vi "Host.vi"() -> ()   [LabVIEW 2025]
uses:
  <vilib>/FPGAPlugInAG/cRIO-9033/niLvFpga_Open_cRIO-9033.vi
  <vilib>/rvi/interface/common/dynamic/niFpgaDynamicAddResources.vi
  <vilib>/FPGAPlugInAG/Dynamic/niLvFpga_Reset_Dynamic.vi
  <vilib>/Utility/error.llb/Error Cluster From Error Code.vi
  <vilib>/rvi/errors/niLvFpgaAdjustHostInterfaceError.vi
  <vilib>/FPGAPlugInAG/Dynamic/niLvFpga_Run_Dynamic.vi
  <vilib>/FPGAPlugInAG/Dynamic/niLvFpga_Close_Dynamic.vi
  <vilib>/rvi/interface/nirviOpenFPGA/nirviOpenFPGA.xnode
  FPGA Bitfiles/parallelhmmlponf_FPGATarget_Target4_-PQN8YsI7Fc.lvbitx
  Target4.vi
  <vilib>/rvi/interface/nirviMethod/nirviMethod.xnode
  <vilib>/rvi/interface/nirviCloseFPGA/nirviCloseFPGA.xnode
  <vilib>/rvi/errors/niLvFpgaMergeErrorWithErrorCode.vi
  <vilib>/FPGAPlugInAG/Dynamic/niLvFpga_ReadFifo_Dynamic.vi
  <vilib>/FPGAPlugInAG/Dynamic/niLvFpga_WriteFifo_Dynamic.vi
panel:
  out "Window(s)":dbl[][](array[numeric])
  out "input":dbl[][](array[numeric])
  out "Healthy%":sgl[](array[numeric])
  out "Unhealthy%":sgl[](array[numeric])
  out "Timing":u32[](array[numeric])
  out "size(s)":i32[](array[numeric])
  out "Uncontrolled Acceleration":dynamicdata(graph)
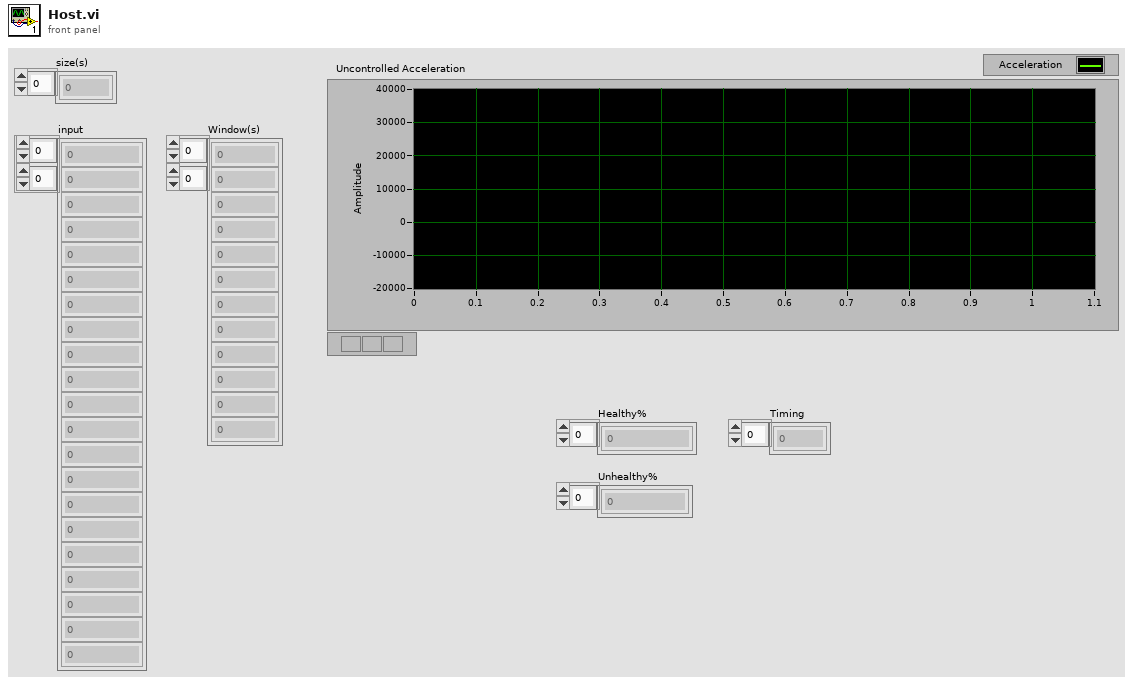
[diagram p1: front panel]
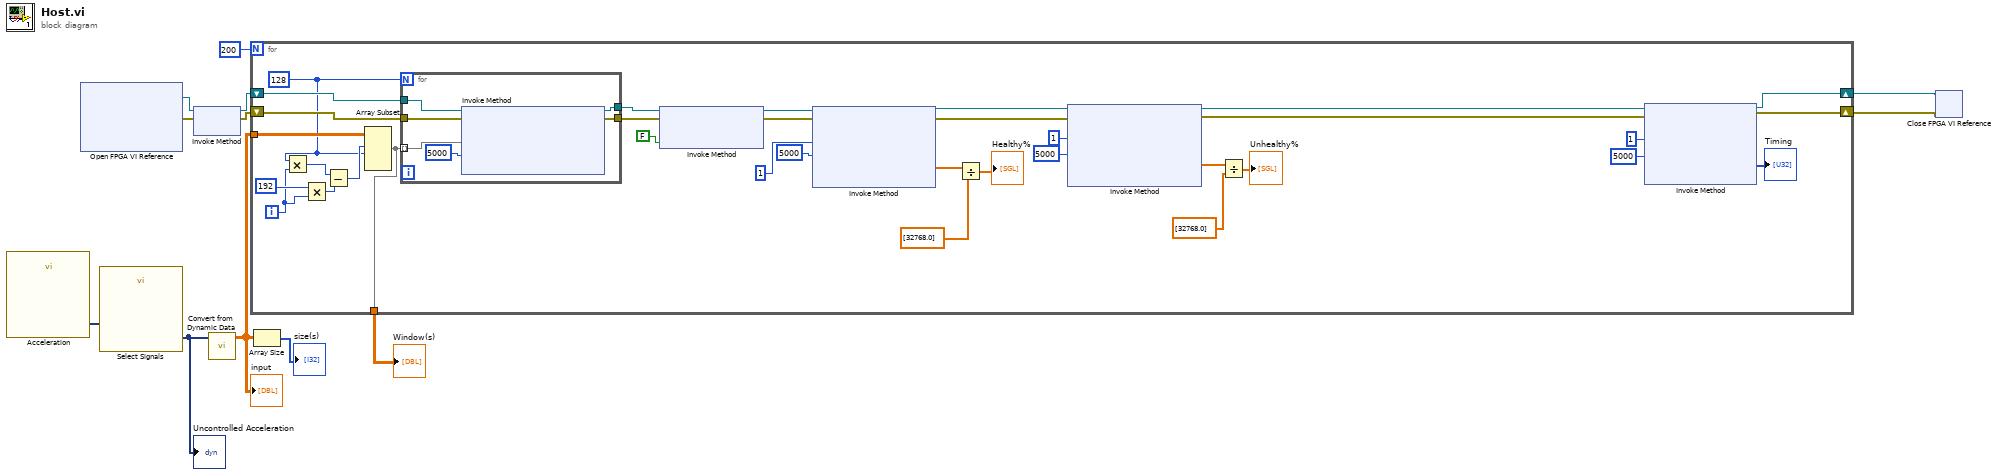
[diagram p0: block diagram]
diagram:
  n1 = call "Acceleration"() -> ("Signals"=w12:dynamicdata)  [unwired: 6 in, 5 out]
  n2 = xnode "Open FPGA VI Reference"() -> ("FPGA VI Reference Out"=w11:refnum<k20>, "error out"=w8:errorcluster)  [unwired: 2 in]
  n3 = call "Select Signals"("Signals"=w12) -> ("Signal Out"=w7:dynamicdata)  [unwired: 9 in, 1 out]
  "Uncontrolled Acceleration" <- w7
  n4 = xnode "Invoke Method"("FPGA VI Reference In"=w11, "error in"=w8) -> ("FPGA VI Reference Out"=w10:refnum<k20>, "error out"=w9:errorcluster)
  n5 = call "Convert from Dynamic Data"("Dynamic Data Type"=w7) -> ("Array"=w2:dbl[][])  [unwired: 3 in]
  "input" <- w2
  n6 = for {
    N: 200 -> [_]
    shift-right: [w16] -> w5
    shift-left: w10 -> [w46]
    shift-right: [w15] -> w4
    shift-left: w9 -> [w45]
    tunnel: w2 -> [w37]
    tunnel: [w36] -> w1
    i -> [w32]
    w30 = 128
    n7 = Multiply(x=w30, y=w32) -> (x*y=w35:i32)
    n8 = Multiply(x=192 ("y"), y=w32) -> (x*y=w31:i32)
    n9 = Subtract(x=w35, y=w31) -> (x-y=w34:i32)
    n10 = Array Subset(array=w37, index (row)=w34, length (row)=w30) -> (w36:dbl[][])  [unwired: 2 in]
    n11 = for {
      N: w30 -> [_]
      tunnel: w46 -> [w52]
      tunnel: w45 -> [w51]
      tunnel: [w49] -> w41
      tunnel: [w48] -> w40
      tunnel: w36 -> [w47] mode=indexing
      n12 = xnode "Invoke Method"("FPGA VI Reference In"=w52, "error in"=w51, "Data"=w47, "Timeout (ms)"=5000) -> ("FPGA VI Reference Out"=w49:refnum<k20>, "error out"=w48:errorcluster)  [unwired: 1 out]
    }
    n13 = xnode "Invoke Method"("FPGA VI Reference In"=w41, "error in"=w40, "Wait Until Done (F)"=FALSE) -> ("FPGA VI Reference Out"=w43:refnum<k20>, "error out"=w42:errorcluster)
    n14 = xnode "Invoke Method"("FPGA VI Reference In"=w43, "error in"=w42, "Number of Elements"=u32 1, "Timeout (ms)"=5000) -> ("FPGA VI Reference Out"=w29:refnum<k20>, "error out"=w28:errorcluster, "Data"=w24:sgl[])  [unwired: 1 out]
    n15 = Divide(x=w24, y=sgl[] [32768.0]) -> (x/y=→"Healthy%":sgl[])
    n16 = xnode "Invoke Method"("FPGA VI Reference In"=w29, "error in"=w28, "Number of Elements"=u32 1, "Timeout (ms)"=5000) -> ("FPGA VI Reference Out"=w14:refnum<k20>, "error out"=w13:errorcluster, "Data"=w21:sgl[])  [unwired: 1 out]
    n17 = Divide(x=w21, y=sgl[] [32768.0]) -> (x/y=→"Unhealthy%":sgl[])
    n18 = xnode "Invoke Method"("FPGA VI Reference In"=w14, "error in"=w13, "Number of Elements"=u32 1, "Timeout (ms)"=5000) -> ("FPGA VI Reference Out"=w16:refnum<k20>, "error out"=w15:errorcluster, "Data"=→"Timing":u32[])  [unwired: 1 out]
  }
  "Window(s)" <- w1
  n19 = Array Size(array=w2) -> (size(s)=→"size(s)":i32[])
  n20 = xnode "Close FPGA VI Reference"("FPGA VI Reference In"=w5, "error in"=w4) -> ()  [unwired: 1 out]
